vi "GetURLandRoot.vi"(10 "?":T1) -> (1 "API root":string, 2 "Base URL":string)   [LabVIEW 2019, in "ByteQXWebAPI.lvlib" / "ByteQXAPIBase.lvclass"]
uses:
  ByteQXAPIBase.lvclass
  module.ctl
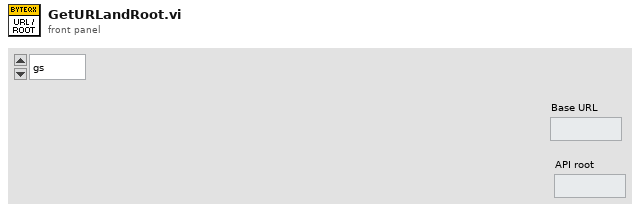
[diagram p1: front panel]
types:
  T1 = typedef "ByteQXWebAPI.lvlib/ByteQXAPIBase.lvclass/module.ctl" = enum16{"gs", "tms"}
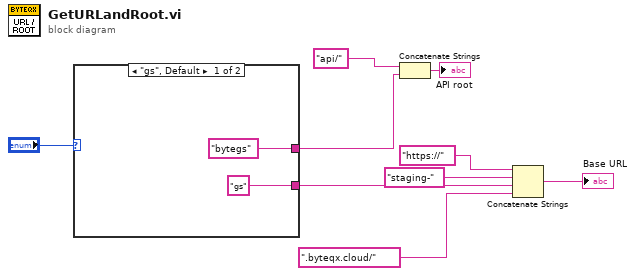
[diagram p0: block diagram]
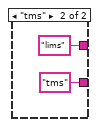
[diagram p2: hidden frame]
diagram:
  n1 = case shown="\"gs\", Default" "?" {
    tunnel: ["bytegs" ("string") "lims" ("string")] -> w8
    tunnel: ["gs" ("string") "tms" ("string")] -> w2
    frame "gs", Default {
    }
    frame "tms" {
    }
  }
  n2 = Concatenate Strings("api/", w8) -> (→"API root":string)
  n3 = Concatenate Strings("https://", "staging-" ("string"), w2, ".byteqx.cloud/" ("string")) -> (→"Base URL":string)
